vi "Send.vi"(5 "Sender":string, 6 "Priority (F)":bool, 7 "Process Name":string, 8 "error in (no error)":errorcluster, 9 "Data":variant, 10 "Message":string) -> (0 "error out":errorcluster)   [LabVIEW 2016, in "System.lvlib"]
uses:
  System.lvlib
  Controls/Control_Message Data.ctl
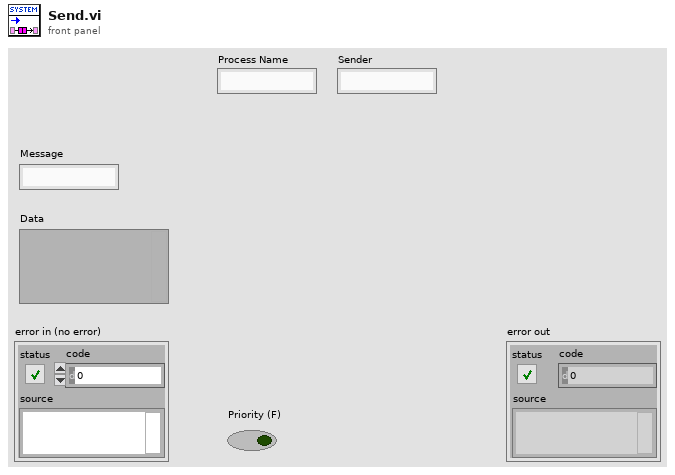
[diagram p1: front panel]
types:
  T1 = typedef "System.lvlib/Control_Message Data.ctl" = cluster{"Message":string, "Data":variant, "Sender":string}
  T2 = typedef "System.lvlib/Control_Variant Data Reference.ctl" = refnum<data-value>
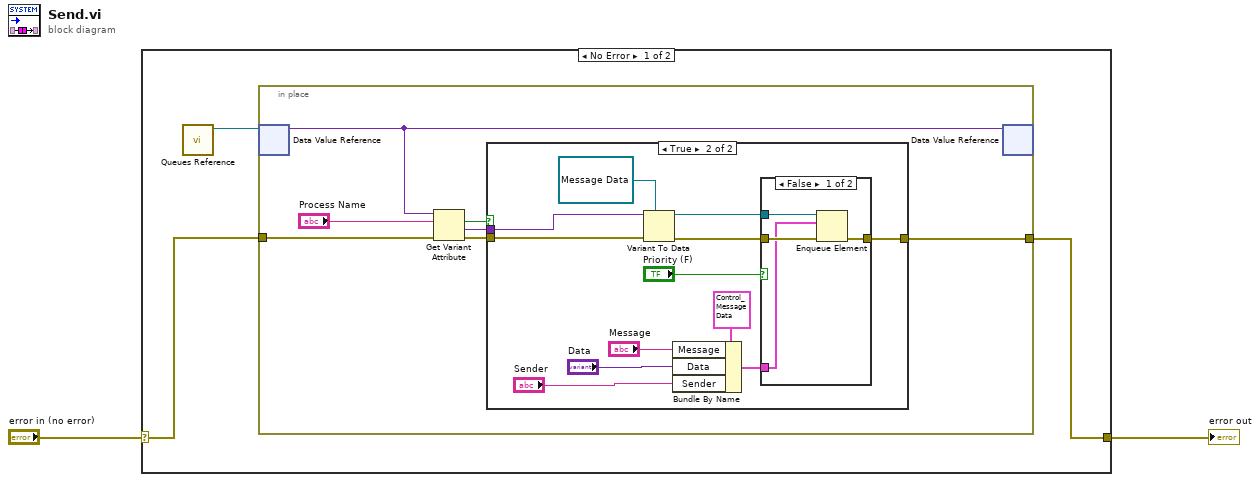
[diagram p0: block diagram]
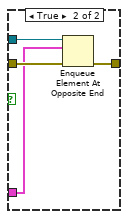
[diagram p3: hidden frame]
diagram:
  n1 = case shown="No Error" "error in (no error)" {
    selector: "error in (no error)" -> [w4 w34]
    tunnel: [w3 w34] -> w1
    frame No Error {
      n2 = call "Queues Reference.vi"() -> ("Queues Reference"=w5:T2)  [unwired: 10 in, 1 out]
      n3 = in-place {
        in-place-border: w4 -> [w8]
        in-place-border: [w7] -> w3
        n4 = in-place-dvr #1(w5) -> (w6:variant)  [unwired: 1 out]
        n5 = Get Variant Attribute(Variant=w6, name="Process Name", error in=w8) -> (found=w11:bool, value=w9:variant, error out=w10:errorcluster)  [unwired: 1 in, 1 out]
        n6 = case shown="True" w11 {
          tunnel: w10 -> [w13 w25]
          tunnel: w9 -> [_ w15]
          tunnel: [w13 w21] -> w7
          frame False {
          }
          frame True {
            n7 = Variant To Data(error in=w25, type=refnum<queue> refnum ("queue out"), Variant=w15) -> (data=w22:refnum<queue>, error out=w23:errorcluster)
            n8 = Bundle By Name(cluster=T1 {"Message"="", "Data"=variant, "Sender"=""} ("Message Data"), "Message"="Message", "Data"="Data", "Sender"="Sender") -> (w18:T1)
            n9 = case shown="False" "Priority (F)" {
              tunnel: w23 -> [w28 w33]
              tunnel: w22 -> [w29 w32]
              tunnel: [w27 w31] -> w21
              tunnel: w18 -> [w26 w30]
              frame False {
                n10 = Enqueue Element(queue=w29, element=w26, error in (no error)=w28) -> (error out=w27:errorcluster)  [unwired: 1 in, 2 out]
              }
              frame True {
                n11 = Enqueue Element At Opposite End(queue=w32, element=w30, error in (no error)=w33) -> (error out=w31:errorcluster)  [unwired: 1 in, 2 out]
              }
            }
          }
        }
        n12 = in-place-dvr #1(w6) -> ()  [unwired: 2 out]
      }
    }
    frame Error {
    }
  }
  "error out" <- w1
